vi "Exemple d'utilisation simple - Valve.vi"() -> ()   [LabVIEW 2013]
panel:
  in  "Valve 5":bool=TRUE
  in  "Valve 4":bool=TRUE
  in  "Valve 3":bool=TRUE
  in  "Valve 2":bool=TRUE
  in  "Valve 1":bool=TRUE
  in  "Stop":bool=TRUE
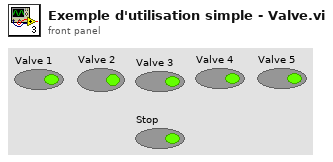
[diagram p1: front panel]
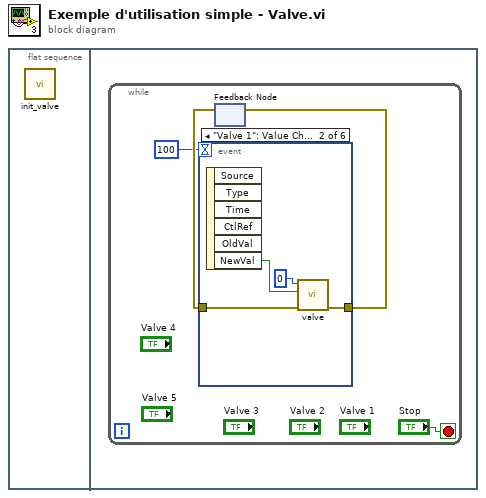
[diagram p0: block diagram]
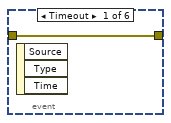
[diagram p2: hidden frame]
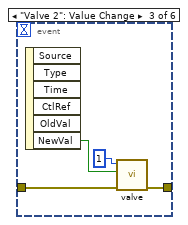
[diagram p3: hidden frame]
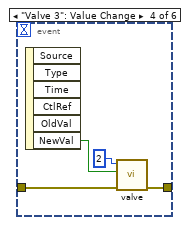
[diagram p4: hidden frame]
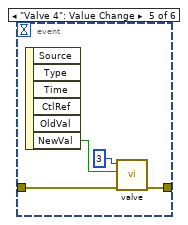
[diagram p5: hidden frame]
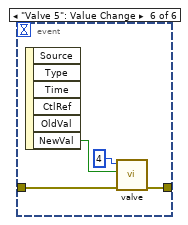
[diagram p6: hidden frame]
diagram:
  n1 = flat-sequence {
    frame #0 {
      n2 = call "init_valve.vi"() -> ()  [unwired: 11 in, 1 out]
    }
    frame #1 {
      n3 = while {
        stop <- "Stop" stop-if-true
        n4 = feedback #1() -> (w2:errorcluster)  [unwired: 1 in]
        n5 = event shown="[1] \"Valve 1\": Value Change" {
          selector: _ -> [_ _ _ _ _ _]
          dyn-events: _ -> [_ _ _ _ _ _]
          timeout: 100 -> [_ _ _ _ _ _]
          tunnel: w2 -> [w5 w8 w12 w16 w20 w24]
          tunnel: [w5 w7 w11 w15 w19 w23] -> w3
          event Timeout {
            n6 = event-data() -> ()  [unwired: 1 in, 3 out]
          }
          event "Valve 1": Value Change {
            n7 = event-data() -> ("NewVal"=w9:bool)  [unwired: 1 in, 5 out]
            n8 = call "valve.vi"("error in"=w8, "ON"=w9, "Valve"=0) -> ("error out"=w7:errorcluster)  [unwired: 8 in]
          }
          event "Valve 2": Value Change {
            n9 = event-data() -> ("NewVal"=w13:bool)  [unwired: 1 in, 5 out]
            n10 = call "valve.vi"("error in"=w12, "ON"=w13, "Valve"=1) -> ("error out"=w11:errorcluster)  [unwired: 8 in]
          }
          event "Valve 3": Value Change {
            n11 = event-data() -> ("NewVal"=w17:bool)  [unwired: 1 in, 5 out]
            n12 = call "valve.vi"("error in"=w16, "ON"=w17, "Valve"=2) -> ("error out"=w15:errorcluster)  [unwired: 8 in]
          }
          event "Valve 4": Value Change {
            n13 = event-data() -> ("NewVal"=w21:bool)  [unwired: 1 in, 5 out]
            n14 = call "valve.vi"("error in"=w20, "ON"=w21, "Valve"=3) -> ("error out"=w19:errorcluster)  [unwired: 8 in]
          }
          event "Valve 5": Value Change {
            n15 = event-data() -> ("NewVal"=w25:bool)  [unwired: 1 in, 5 out]
            n16 = call "valve.vi"("error in"=w24, "ON"=w25, "Valve"=4) -> ("error out"=w23:errorcluster)  [unwired: 8 in]
          }
        }
        n17 = feedback-in #1(w3) -> ()
      }
    }
  }
